vi "Find While Loop from Structure.vi"(8 "error in (no error)":errorcluster, 11 "MultiFrameStructure in":refnum<vi>) -> (0 "error out":errorcluster, 3 "WLoop Refnum":refnum<vi>)   [LabVIEW 2020, in "JKI State Machine API.lvlib" / "JKI SM.lvclass"]
uses:
  JKI SM.lvclass
  JKI SM.lvclass/JKI SM.ctl
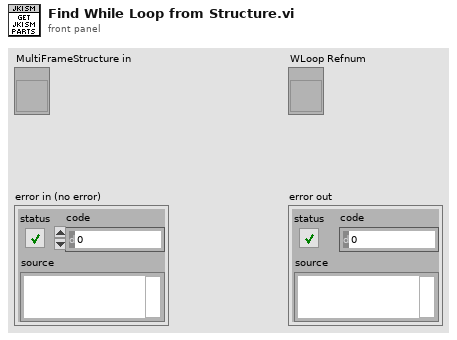
[diagram p1: front panel]
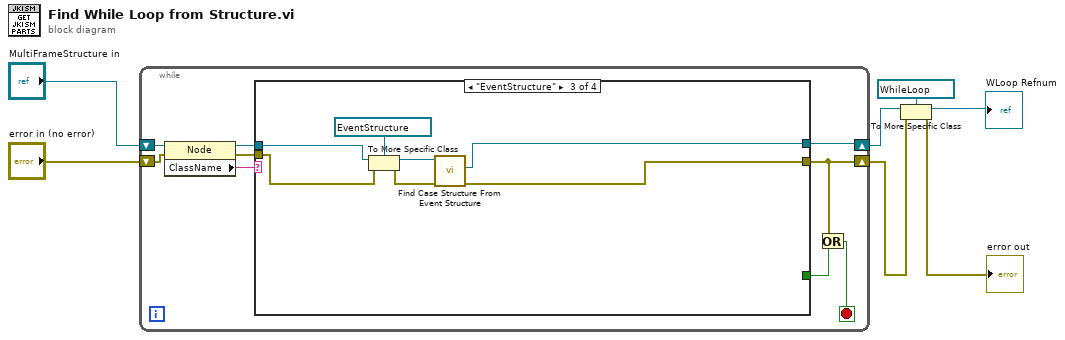
[diagram p0: block diagram]
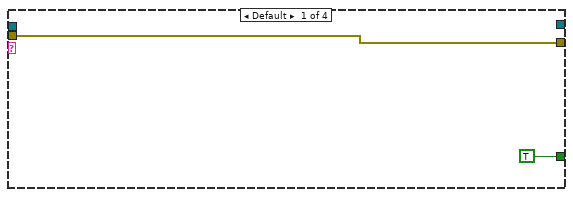
[diagram p2: hidden frame]
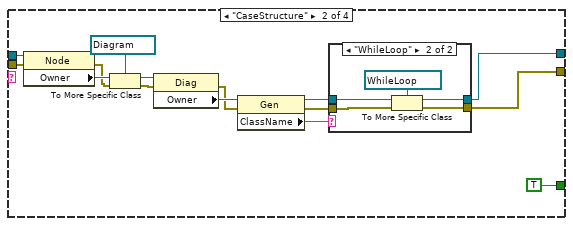
[diagram p3: hidden frame]
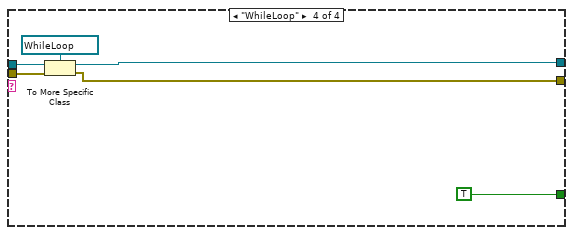
[diagram p5: hidden frame]
diagram:
  n1 = while {
    shift-right: [w12] -> w4
    shift-left: "MultiFrameStructure in" -> [w16]
    shift-right: [w10] -> w2
    shift-left: "error in (no error)" -> [w11]
    stop <- w9 stop-if-true
    n2 = property class="Node"(reference=w16, error in=w11) -> (reference out=w14:refnum<vi>, error out=w13:errorcluster, "ClassName"=w15:string)
    n3 = case shown="\"EventStructure\"" w15 {
      tunnel: w14 -> [_ w33 w44 w52]
      tunnel: w13 -> [w17 w32 w41 w51]
      tunnel: [_ w21 w45 w48] -> w12
      tunnel: [w17 w20 w46 w49] -> w10
      tunnel: [TRUE TRUE _ TRUE] -> w8
      frame Default {
      }
      frame "CaseStructure" {
        n4 = property class="Node"(reference=w33, error in=w32) -> (error out=w28:errorcluster, "Owner"=w31:refnum<vi>)  [unwired: 1 out]
        n5 = To More Specific Class(target class=refnum<vi> refnum ("Diag Refnum"), reference=w31, error in=w28) -> (specific class reference=w27:refnum<vi>, error out=w29:errorcluster)
        n6 = property class="Diag"(reference=w27, error in=w29) -> (error out=w22:errorcluster, "Owner"=w23:refnum<vi>)  [unwired: 1 out]
        n7 = property class="Gen"(reference=w23, error in=w22) -> (reference out=w26:refnum<vi>, error out=w25:errorcluster, "ClassName"=w24:string)
        n8 = case shown="\"WhileLoop\"" w24 {
          tunnel: [_ w39] -> w21
          tunnel: [w34 w38] -> w20
          tunnel: w26 -> [_ w37]
          tunnel: w25 -> [w34 w36]
          frame Default {
          }
          frame "WhileLoop" {
            n9 = To More Specific Class(target class=refnum<vi> refnum ("WLoop Refnum"), reference=w37, error in=w36) -> (specific class reference=w39:refnum<vi>, error out=w38:errorcluster)
          }
        }
      }
      frame "EventStructure" {
        n10 = To More Specific Class(target class=refnum<vi> refnum ("EvntStruct Refnum"), reference=w44, error in=w41) -> (specific class reference=w43:refnum<vi>, error out=w40:errorcluster)
        n11 = call "Find Case Structure From Event Structure.vi"("error in (no error)"=w40, "EvntStruct Refnum"=w43) -> ("error out"=w46:errorcluster, "CaseStructure out"=w45:refnum<vi>)  [unwired: 8 in]
      }
      frame "WhileLoop" {
        n12 = To More Specific Class(target class=refnum<vi> refnum ("WLoop Refnum"), reference=w52, error in=w51) -> (specific class reference=w48:refnum<vi>, error out=w49:errorcluster)
      }
    }
    n13 = Or(x=w10, y=w8) -> (x .or. y?=w9:bool)
  }
  n14 = To More Specific Class(target class=refnum<vi> refnum ("WLoop Refnum"), reference=w4, error in=w2) -> (specific class reference=→"WLoop Refnum":refnum<vi>, error out=→"error out":errorcluster)
